vi "Datas2Bytes.vi"(10 "DATAs":string) -> (0 "Data5":u32, 1 "Data4":u32, 2 "Data3":u32, 3 "Data2":u32, 4 "Data6":u32, 5 "Data1":u32, 6 "Data7":u32, 7 "Data0":u32)   [LabVIEW 2015]
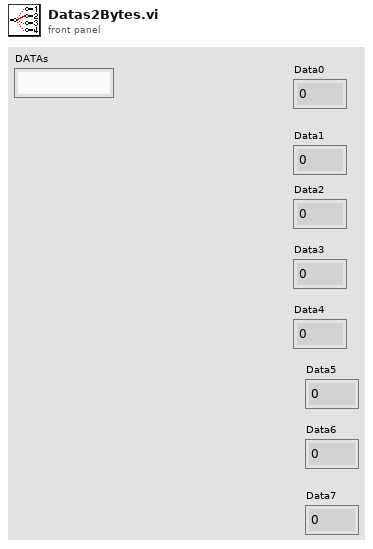
[diagram p1: front panel]
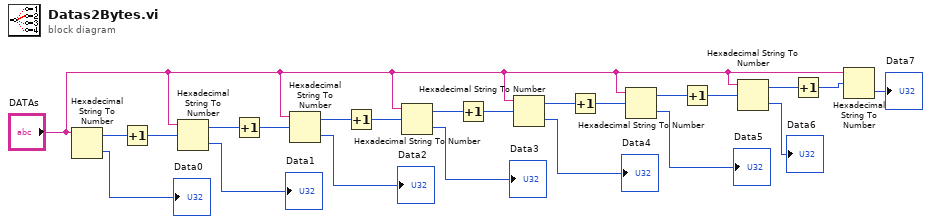
[diagram p0: block diagram]
diagram:
  n1 = Hexadecimal String To Number(string="DATAs") -> (offset past number=w2:i32, number=→"Data0":u32)  [unwired: 2 in]
  n2 = Increment(x=w2) -> (x+1=w1:i32)
  n3 = Hexadecimal String To Number(string="DATAs", offset=w1) -> (offset past number=w6:i32, number=→"Data1":u32)  [unwired: 1 in]
  n4 = Increment(x=w6) -> (x+1=w5:i32)
  n5 = Hexadecimal String To Number(string="DATAs", offset=w5) -> (offset past number=w3:i32, number=→"Data2":u32)  [unwired: 1 in]
  n6 = Increment(x=w3) -> (x+1=w4:i32)
  n7 = Hexadecimal String To Number(string="DATAs", offset=w4) -> (offset past number=w14:i32, number=→"Data3":u32)  [unwired: 1 in]
  n8 = Increment(x=w14) -> (x+1=w13:i32)
  n9 = Hexadecimal String To Number(string="DATAs", offset=w13) -> (offset past number=w11:i32, number=→"Data4":u32)  [unwired: 1 in]
  n10 = Increment(x=w11) -> (x+1=w12:i32)
  n11 = Hexadecimal String To Number(string="DATAs", offset=w12) -> (offset past number=w7:i32, number=→"Data5":u32)  [unwired: 1 in]
  n12 = Increment(x=w7) -> (x+1=w8:i32)
  n13 = Hexadecimal String To Number(string="DATAs", offset=w8) -> (offset past number=w10:i32, number=→"Data6":u32)  [unwired: 1 in]
  n14 = Increment(x=w10) -> (x+1=w9:i32)
  n15 = Hexadecimal String To Number(string="DATAs", offset=w9) -> (number=→"Data7":u32)  [unwired: 1 in, 1 out]
